vi "HEALTH_LABVIEW_V6.vi"() -> ()   [LabVIEW 2026]
uses:
  <vilib>/addons/control/pid/pid.llb/PID (DBL).vi
  <vilib>/addons/control/pid/NI_PID_pid.lvlib
panel:
  in  "CLEAR GRAPHS":bool
  in  "TEMP SENSOR\nZEROING VALUE (C)":dbl
  in  "FLOW PID gains":T1={"proportional gain (Kc)"=1.0, "integral time (Ti, min)"=0.01, "derivative time (Td, min)"=0.0} {"derivative time (Td, min)" format="%.3f"; "integral time (Ti, min)" format="%.3f"; "proportional gain (Kc)" format="%.3f"}
  in  "TARGET FLOW RATE (LPM)":dbl format="%.2f"
  in  "HEATER PID gains":T1={"proportional gain (Kc)"=1.0, "integral time (Ti, min)"=0.01, "derivative time (Td, min)"=0.0} {"derivative time (Td, min)" format="%.3f"; "integral time (Ti, min)" format="%.3f"; "proportional gain (Kc)" format="%.3f"}
  out "HEATER SIDE BLOCK RTD":dbl(graph)
  out "OUTLET TEMP (C)":dbl format="%#_3g"
  out "INLET TEMP (C)":dbl format="%#_3g"
  out "INLET PRESSURE (PSI)":dbl(graph)
  out "PRESSURE DROP (PSI)":dbl(graph)
  out "DELTA T (C)":dbl format="%#_3f"
  out "DELTA T (C)":dbl(graph)
  out "COOLANT FLOW RATE":dbl(graph)
  in  "PUMP ON/OFF":bool
  out "HX SIDE BLOCK RTD":cluster{dbl, "TARGET HX TEMP (C)":dbl}(graph)
  out "HEATER POWER OUTPUT":dbl(knob) scale=0.0..100.0
  in  "TARGET HX TEMP (C)":dbl
  in  "HEATER ON/OFF":bool
  in  "stop":bool
  out "Error String":string
  out "error out":errorcluster
  out "ConnectionType Out":i32
  out "DeviceType Out":i32
  in  "Identifier":string="LJM_idANY"
  in  "ConnectionType":string="LJM_ctANY"
  in  "DeviceType":string="LJM_dtANY"
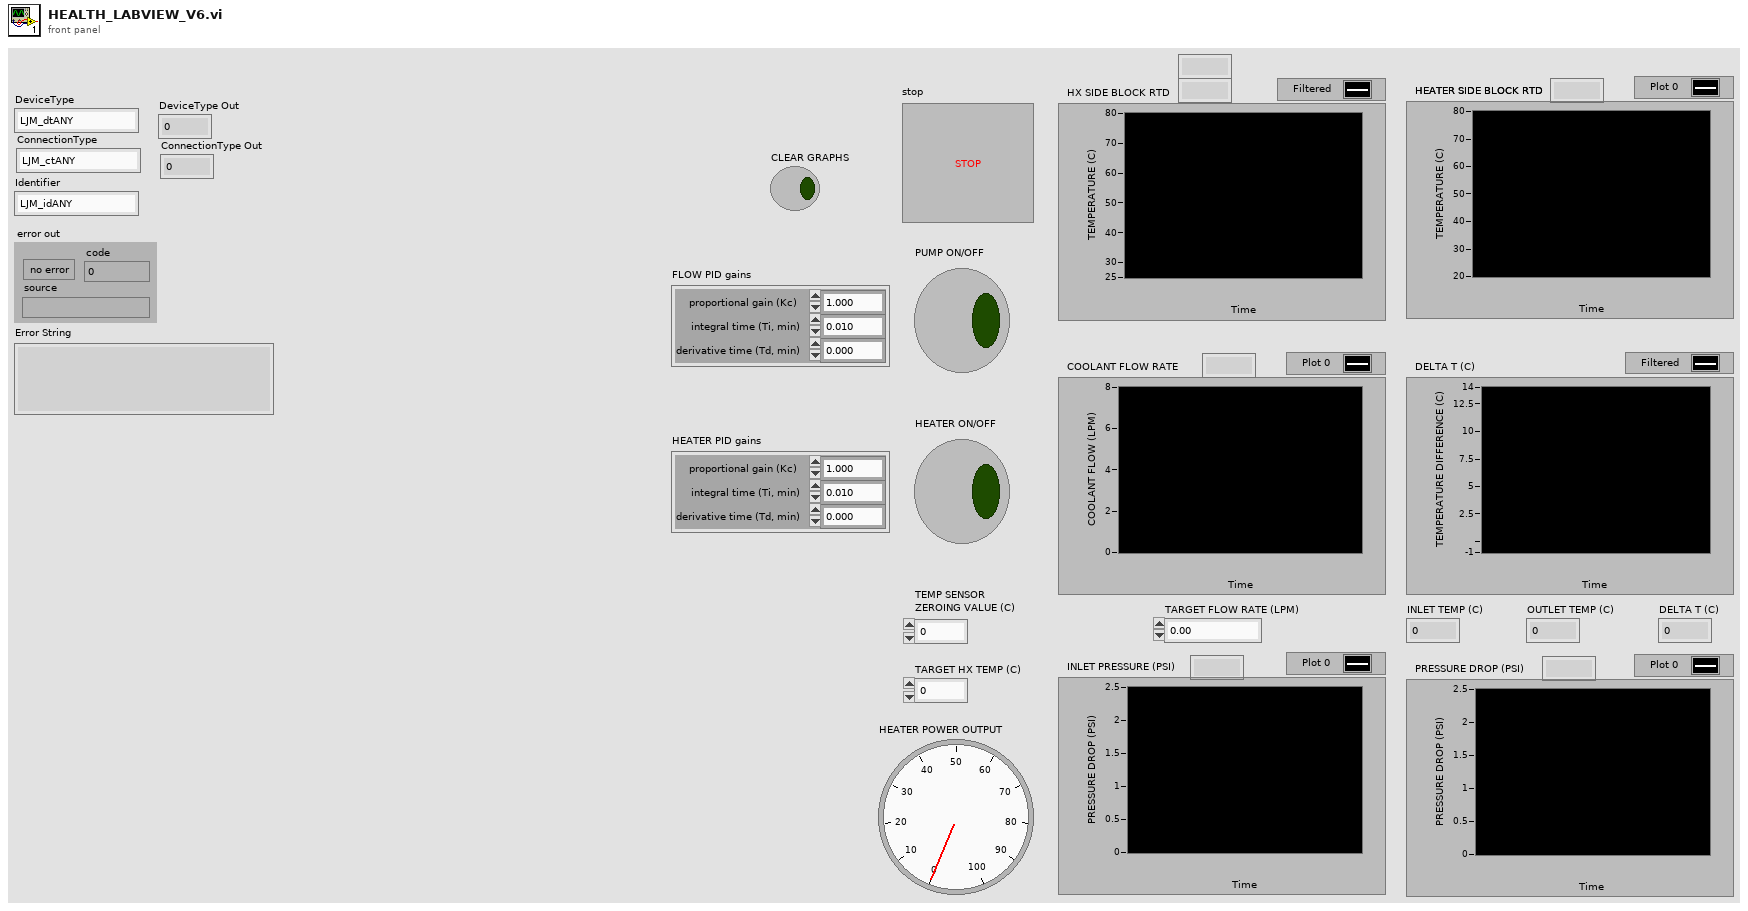
[diagram p1: front panel]
types:
  T1 = cluster{"proportional gain (Kc)":dbl, "integral time (Ti, min)":dbl, "derivative time (Td, min)":dbl}
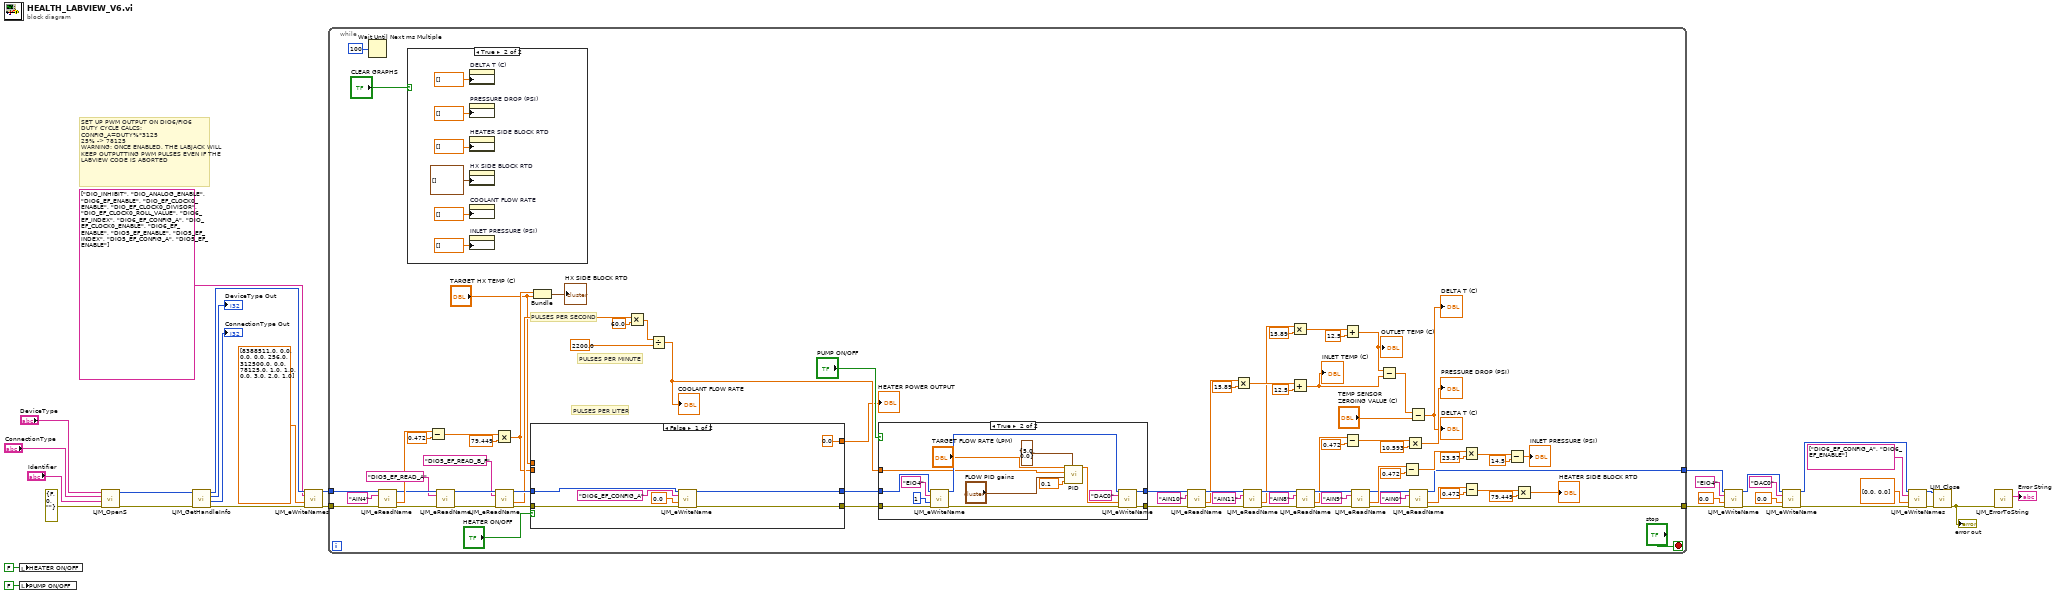
[diagram p0: block diagram]
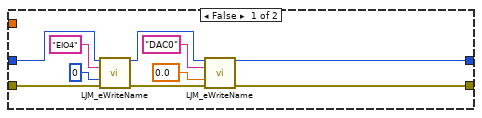
[diagram p3: hidden frame]
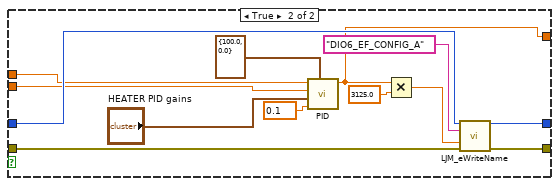
[diagram p4: hidden frame]
diagram:
  # "SET UP PWM OUTPUT ON DIO6/FIO6\nDUTY CYCLE CALCS:\nCONFIG_A=DUTY%*3125\n25% -> 78125\nWARNING: ONCE ENABLED, THE LABJACK WILL KEEP OUTPUTTING PWM PULSES EVEN IF THE LABVIEW CODE IS ABORTED"
  n1 = local write "HEATER ON/OFF"(FALSE ("HEATER ON/OFF 2")) -> ()
  n2 = local write "PUMP ON/OFF"(FALSE ("PUMP ON/OFF 2")) -> ()
  n3 = call "LJM_OpenS.vi"("error in"=errorcluster {"status"=FALSE, "code"=0, "source"=""} ("error in (no error)"), "Identifier"="Identifier", "ConnectionType"="ConnectionType", "DeviceType"="DeviceType") -> ("error out"=w31:errorcluster, "Handle"=w30:i32)  [unwired: 6 in]
  n4 = call "LJM_GetHandleInfo.vi"("error in"=w31, "Handle In"=w30) -> ("error out"=w21:errorcluster, "ConnectionType"=→"ConnectionType Out":i32, "DeviceType"=→"DeviceType Out":i32, "Handle Out"=w22:i32)  [unwired: 2 in, 4 out]
  n5 = call "LJM_eWriteNames.vi"("Handle In"=w22, "aNames"=string[] ["DIO_INHIBIT", "DIO_ANALOG_ENABLE", "DIO6_EF_ENABLE", "DIO_EF_CLOCK0_ENABLE", "DIO_EF_CLOCK0_DIVISOR", "DIO_EF_CLOCK0_ROLL_VALUE", "DIO6_EF_INDEX", "DIO6_EF_CONFIG_A", "DIO_EF_CLOCK0_ENABLE", "DIO6_EF_ENABLE", "DIO5_EF_ENABLE", "DIO5_EF_INDEX", "DIO5_EF_CONFIG_A", "DIO5_EF_ENABLE"], "aValuesIn"=dbl[] [8388511.0, 0.0, 0.0, 0.0, 256.0, 312500.0, 0.0, 78125.0, 1.0, 1.0, 0.0, 3.0, 2.0, 1.0], "error in"=w21) -> ("Handle Out"=w2:i32, "error out"=w1:errorcluster)  [unwired: 9 in, 1 out]
  n6 = while {
    tunnel: [w57] -> w9
    tunnel: w2 -> [w100]
    tunnel: w1 -> [w99]
    tunnel: [w58] -> w3
    stop <- "stop" stop-if-true
    # "PULSES PER LITER"
    # "PULSES PER MINUTE"
    # "PULSES PER SECOND"
    n7 = Wait Until Next ms Multiple(millisecond multiple=u32 100 ("milliseconds to wait")) -> ()  [unwired: 1 out]
    n8 = call "LJM_eReadName.vi"("Handle In"=w100, "Name"="AIN4", "error in"=w99) -> ("Handle Out"=w98:i32, "Value"=w106:dbl, "error out"=w97:errorcluster)  [unwired: 10 in]
    n9 = case shown="True" "CLEAR GRAPHS" {
      frame False {
      }
      frame True {
        n10 = property on="DELTA T (C)" class="WFChart (strict)"("History Data"=dbl[] []) -> ()  [unwired: 2 in, 2 out]
        n11 = property on="PRESSURE DROP (PSI)" class="WFChart (strict)"("History Data"=dbl[] []) -> ()  [unwired: 2 in, 2 out]
        n12 = property on="HEATER SIDE BLOCK RTD" class="WFChart (strict)"("History Data"=dbl[] []) -> ()  [unwired: 2 in, 2 out]
        n13 = property on="HX SIDE BLOCK RTD" class="WFChart (strict)"("History Data"=cluster{dbl, "TARGET HX TEMP (C)":dbl}[] []) -> ()  [unwired: 2 in, 2 out]
        n14 = property on="COOLANT FLOW RATE" class="WFChart (strict)"("History Data"=dbl[] []) -> ()  [unwired: 2 in, 2 out]
        n15 = property on="INLET PRESSURE (PSI)" class="WFChart (strict)"("History Data"=dbl[] []) -> ()  [unwired: 2 in, 2 out]
      }
    }
    n16 = Subtract(x=w106, y=0.472 ("Address 2")) -> (x-y=w109:dbl)
    n17 = call "LJM_eReadName.vi"("Handle In"=w98, "Name"="DIO5_EF_READ_A", "error in"=w97) -> ("Handle Out"=w95:i32, "error out"=w92:errorcluster)  [unwired: 10 in, 1 out]
    n18 = Multiply(x=w109, y=79.449 ("Address 2")) -> (x*y=w36:dbl)
    n19 = call "LJM_eReadName.vi"("Handle In"=w95, "Name"="DIO5_EF_READ_B_F" ("DIO5_EF_READ_B_F"), "error in"=w92) -> ("Handle Out"=w94:i32, "Value"=w51:dbl, "error out"=w93:errorcluster)  [unwired: 10 in]
    n20 = case shown="False" "HEATER ON/OFF" {
      tunnel: [w147 w161] -> w101
      tunnel: [w148 w160] -> w102
      tunnel: "TARGET HX TEMP (C)" -> [_ w153]
      tunnel: w36 -> [_ w154]
      tunnel: w94 -> [w144 w156]
      tunnel: w93 -> [w143 w155]
      tunnel: [0.0 ("output") w149] -> w34
      frame False {
        n21 = call "LJM_eWriteName.vi"("Handle In"=w144, "Name"="DIO6_EF_CONFIG_A", "Value"=0.0, "error in"=w143) -> ("Handle Out"=w148:i32, "error out"=w147:errorcluster)  [unwired: 10 in]
      }
      frame True {
        n22 = call-poly <vilib>:"PID.vi"("output range"=cluster{"output high":dbl, "output low":dbl} {"output high"=100.0, "output low"=0.0}, "dt (s)"=0.1, "PID gains"="HEATER PID gains", "process variable"=w154, "setpoint"=w153) -> ("output"=w149:dbl)  [unwired: 5 in, 1 out]
        n23 = Multiply(x=w149, y=3125.0) -> (x*y=w158:dbl)
        n24 = call "LJM_eWriteName.vi"("Handle In"=w156, "Name"="DIO6_EF_CONFIG_A", "Value"=w158, "error in"=w155) -> ("Handle Out"=w160:i32, "error out"=w161:errorcluster)  [unwired: 10 in]
      }
    }
    "HEATER POWER OUTPUT" <- w34
    n25 = Bundle(w36, "TARGET HX TEMP (C)"="TARGET HX TEMP (C)") -> (→"HX SIDE BLOCK RTD":cluster{dbl, "TARGET HX TEMP (C)":dbl})  [unwired: 1 in]
    n26 = Multiply(x=w51, y=60.0) -> (x*y=w49:dbl)
    n27 = Divide(x=w49, y=2200.0) -> (x/y=w47:dbl)
    "COOLANT FLOW RATE" <- w47
    n28 = case shown="True" "PUMP ON/OFF" {
      tunnel: w102 -> [w124 w139]
      tunnel: w101 -> [w123 w138]
      tunnel: [w119 w133] -> w86
      tunnel: [w118 w134] -> w90
      tunnel: w47 -> [_ w132]
      frame False {
        n29 = call "LJM_eWriteName.vi"("Handle In"=w124, "Name"="EIO4", "Value"=0, "error in"=w123) -> ("Handle Out"=w121:i32, "error out"=w120:errorcluster)  [unwired: 10 in]
        n30 = call "LJM_eWriteName.vi"("Handle In"=w121, "Name"="DAC0", "Value"=0.0, "error in"=w120) -> ("Handle Out"=w118:i32, "error out"=w119:errorcluster)  [unwired: 10 in]
      }
      frame True {
        n31 = call "LJM_eWriteName.vi"("Handle In"=w139, "Name"="EIO4", "Value"=1, "error in"=w138) -> ("Handle Out"=w135:i32, "error out"=w136:errorcluster)  [unwired: 10 in]
        n32 = call-poly <vilib>:"PID.vi"("output range"=cluster{"output high":dbl, "output low":dbl} {"output high"=5.0, "output low"=0.0}, "dt (s)"=0.1 ("FLOW dt (s)"), "PID gains"="FLOW PID gains", "process variable"=w132, "setpoint"="TARGET FLOW RATE (LPM)") -> ("output"=w127:dbl)  [unwired: 5 in, 1 out]
        n33 = call "LJM_eWriteName.vi"("Handle In"=w135, "Name"="DAC0", "Value"=w127, "error in"=w136) -> ("Handle Out"=w134:i32, "error out"=w133:errorcluster)  [unwired: 10 in]
      }
    }
    n34 = call "LJM_eReadName.vi"("Handle In"=w90, "Name"="AIN10", "error in"=w86) -> ("Handle Out"=w89:i32, "Value"=w45:dbl, "error out"=w85:errorcluster)  [unwired: 10 in]
    n35 = Multiply(x=w45, y=15.89) -> (x*y=w77:dbl)
    n36 = call "LJM_eReadName.vi"("Handle In"=w89, "Name"="AIN11" ("Name 2"), "error in"=w85) -> ("Handle Out"=w88:i32, "Value"=w44:dbl, "error out"=w84:errorcluster)  [unwired: 10 in]
    n37 = Multiply(x=w44, y=15.89) -> (x*y=w74:dbl)
    n38 = Add(x=w77, y=12.5) -> (x+y=w42:dbl)
    "INLET TEMP (C)" <- w42
    n39 = call "LJM_eReadName.vi"("Handle In"=w88, "Name"="AIN8" ("Name 3"), "error in"=w84) -> ("Handle Out"=w87:i32, "Value"=w61:dbl, "error out"=w83:errorcluster)  [unwired: 10 in]
    n40 = Add(x=w74, y=12.5) -> (x+y=w43:dbl)
    "OUTLET TEMP (C)" <- w43
    n41 = Subtract(x=w61, y=0.472) -> (x-y=w71:dbl)
    n42 = call "LJM_eReadName.vi"("Handle In"=w87, "Name"="AIN9" ("Name 4"), "error in"=w83) -> ("Handle Out"=w60:i32, "Value"=w65:dbl, "error out"=w59:errorcluster)  [unwired: 10 in]
    n43 = Subtract(x=w43, y=w42) -> (x-y=w41:dbl)
    n44 = Subtract(x=w65, y=0.472) -> (x-y=w67:dbl)
    n45 = Multiply(x=w71, y=10.593) -> (x*y=→"PRESSURE DROP (PSI)":dbl)
    n46 = Subtract(x=w41, y="TEMP SENSOR\nZEROING VALUE (C)") -> (x-y=→"DELTA T (C)" →"DELTA T (C)":dbl)
    n47 = call "LJM_eReadName.vi"("Handle In"=w60, "Name"="AIN0", "error in"=w59) -> ("Handle Out"=w57:i32, "Value"=w52:dbl, "error out"=w58:errorcluster)  [unwired: 10 in]
    n48 = Multiply(x=w67, y=23.57) -> (x*y=w63:dbl)
    n49 = Subtract(x=w52, y=0.472 ("Address 2")) -> (x-y=w55:dbl)
    n50 = Subtract(x=w63, y=14.5) -> (x-y=→"INLET PRESSURE (PSI)":dbl)
    n51 = Multiply(x=w55, y=79.449 ("Address 2")) -> (x*y=→"HEATER SIDE BLOCK RTD":dbl)
  }
  n52 = call "LJM_eWriteName.vi"("Handle In"=w9, "Name"="EIO4", "Value"=0.0, "error in"=w3) -> ("Handle Out"=w10:i32, "error out"=w13:errorcluster)  [unwired: 10 in]
  n53 = call "LJM_eWriteName.vi"("Handle In"=w10, "Name"="DAC0", "Value"=0.0, "error in"=w13) -> ("Handle Out"=w11:i32, "error out"=w12:errorcluster)  [unwired: 10 in]
  n54 = call "LJM_eWriteNames.vi"("Handle In"=w11, "aNames"=string[] ["DIO6_EF_CONFIG_A", "DIO6_EF_ENABLE"], "aValuesIn"=dbl[] [0.0, 0.0], "error in"=w12) -> ("Handle Out"=w17:i32, "error out"=w18:errorcluster)  [unwired: 9 in, 1 out]
  n55 = call "LJM_Close.vi"("error in"=w18, "Handle"=w17) -> ("error out"=w23:errorcluster)  [unwired: 9 in]
  "error out" <- w23
  n56 = call "LJM_ErrorToString.vi"("error in"=w23) -> ("String"=→"Error String":string)  [unwired: 10 in]
